vi "Update Laser Output.vi"(8 "error in":errorcluster, 11 "cPAS in":refnum<class "cPAS.lvclass">) -> (0 "error out":errorcluster, 3 "cPAS out":refnum<class "cPAS.lvclass">)   [LabVIEW 2015, in "cPAS.lvclass"]
uses:
  cPAS.lvclass
  Reusable/PAS/Main/PAS.lvclass
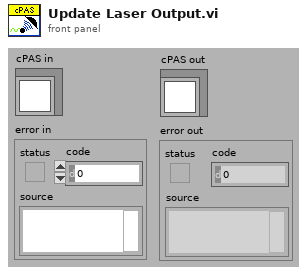
[diagram p1: front panel]
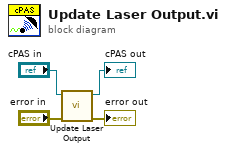
[diagram p0: block diagram]
diagram:
  n1 = call-parent "Update Laser Output.vi"("error in"="error in", "PAS in"="cPAS in") -> ("error out"=→"error out":errorcluster, "PAS out"=→"cPAS out":refnum<class "cPAS.lvclass">)  [unwired: 8 in]
